vi "整体初始化.vi"(8 "错误输入（无错误）":errorcluster, 11 "Scintilla":refnum<k24>) -> (0 "错误输出":errorcluster, 3 "引用输出":refnum<k24>)   [LabVIEW 2018]
uses:
  ScintillaNET.dll
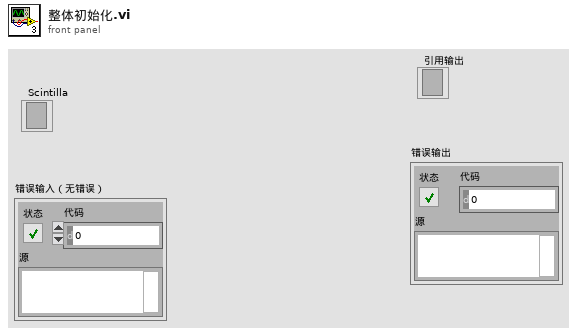
[diagram p1: front panel]
types:
  T1 = cluster{"大小":i32, "粗体":bool, "下划线":bool, "斜体":bool, "背景色":u32, "前景色":u32, "Font":string}
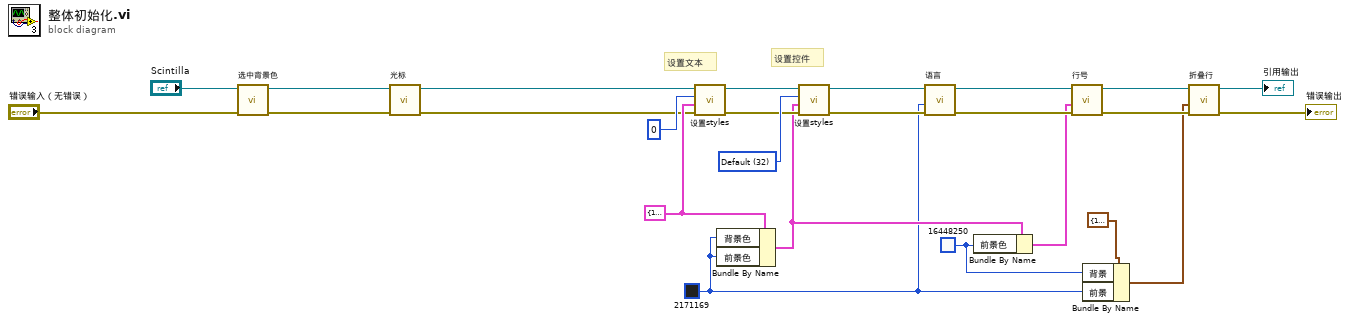
[diagram p0: block diagram]
diagram:
  w6 = u32 16448250 ("前景色")
  w7 = u32 2171169 ("前景色")
  w11 = T1 {"大小"=15, "粗体"=FALSE, "下划线"=FALSE, "斜体"=FALSE, "背景色"=0, "前景色"=0, "Font"=""} ("外观属性")
  w19 = 32 items=["Default"=32, "LineNumber"=33, "BraceLight"=34, "BraceBad"=35, "IndentGuide"=37, "CallTip"=38, "FoldDisaplayText"=39] ("设置项")
  # "设置控件"
  # "设置文本"
  n1 = call "选中背景色.vi"("错误输入（无错误）"="错误输入（无错误）", "引用"="Scintilla") -> ("错误输出"=w2:errorcluster, "引用输出"=w4:refnum<k24>)  [unwired: 8 in]
  n2 = call "光标.vi"("错误输入"=w2, "引用"=w4) -> ("错误输出"=w1:errorcluster, "引用输出"=w3:refnum<k24>)  [unwired: 8 in]
  n3 = call "设置styles.vi"("错误输入（无错误）"=w1, "外观属性"=w11, "设置项"=0, "Scintilla"=w3) -> ("错误输出"=w17:errorcluster, "Scintilla"=w18:refnum<k24>)  [unwired: 6 in]
  n4 = Bundle By Name(cluster=w11, "背景色"=w7, "前景色"=w7) -> (w10:T1)
  n5 = call "设置styles.vi"("错误输入（无错误）"=w17, "外观属性"=w10, "设置项"=w19, "Scintilla"=w18) -> ("错误输出"=w14:errorcluster, "Scintilla"=w15:refnum<k24>)  [unwired: 6 in]
  n6 = call "语言.vi"("错误输入（无错误）"=w14, "背景色"=w7, "Scintilla"=w15) -> ("错误输出"=w12:errorcluster, "Scintilla"=w13:refnum<k24>)  [unwired: 7 in]
  n7 = Bundle By Name(cluster=w10, "前景色"=w6) -> (w9:T1)
  n8 = call "行号.vi"("错误输入（无错误）"=w12, "外观属性"=w9, "Scintilla"=w13) -> ("错误输出"=w20:errorcluster, "引用输出"=w21:refnum<k24>)  [unwired: 7 in]
  n9 = Bundle By Name(cluster=cluster{"背景":u32, "前景":u32} {"背景"=16448250, "前景"=16448250} ("簇"), "背景"=w6, "前景"=w7) -> (w5:cluster{"背景":u32, "前景":u32})
  n10 = call "折叠行.vi"("错误输入（无错误）"=w20, "簇"=w5, "引用"=w21) -> ("错误输出"=→"错误输出":errorcluster, "Scintilla"=→"引用输出":refnum<k24>)  [unwired: 7 in]
